vi "Array Dedup_1D Str.vi"(6 "정렬?":bool, 8 "error in (no error)":errorcluster caption="에러 입력(에러 없음)", 11 "배열 in":string[](array[string])) -> (0 "error out":errorcluster caption="에러 출력", 3 "배열 out":string[](array[string]))   [LabVIEW 2020]
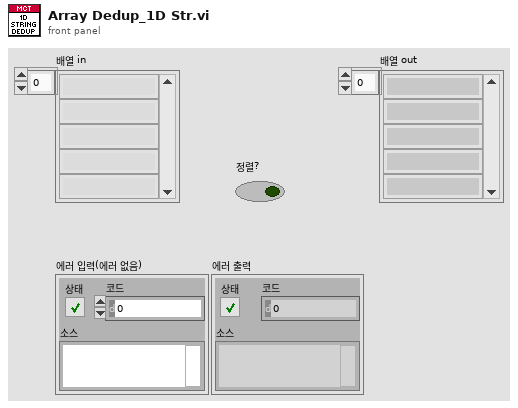
[diagram p1: front panel]
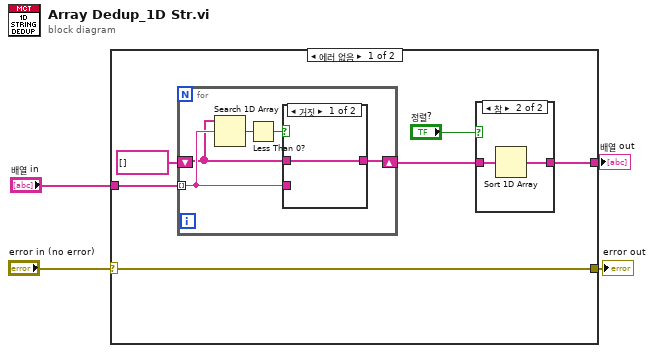
[diagram p0: block diagram]
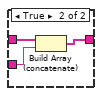
[diagram p3: hidden frame]
diagram:
  n1 = case shown="에러 없음" "error in (no error)" {
    selector: "error in (no error)" -> [w9 w23]
    tunnel: "배열 in" -> [w10 w24]
    tunnel: [w6 w24] -> w3
    tunnel: [w9 w23] -> w1
    frame No Error {
      n2 = for {
        tunnel: w10 -> [w15] mode=indexing
        shift-right: [w16] -> w7
        shift-left: string[] [] -> [w14]
        n3 = Search 1D Array(1D array=w14, element=w15) -> (index of element=w18:i32)  [unwired: 1 in]
        n4 = Less Than 0?(x=w18) -> (x < 0?=w17:bool)
        n5 = case shown="거짓" w17 {
          tunnel: [w19 w22] -> w16
          tunnel: w14 -> [w19 w21]
          tunnel: w15 -> [_ w20]
          frame False {
          }
          frame True {
            n6 = Build Array (concatenate)(w21, w20) -> (w22:string[])
          }
        }
      }
      n7 = case shown="참" "정렬?" {
        tunnel: w7 -> [w11 w13]
        tunnel: [w11 w12] -> w6
        frame False {
        }
        frame True {
          n8 = Sort 1D Array(array=w13) -> (sorted array=w12:string[])
        }
      }
    }
    frame Error {
    }
  }
  "배열 out" <- w3
  "error out" <- w1
